vi "Write numAverages.vi"(8 "error in (no error)":errorcluster, 10 "numAverages":u16, 11 "CaptureSpectImage in":refnum<class "captureSpectImage.lvclass">) -> (0 "error out":errorcluster, 3 "CaptureSpectImage out":refnum<class "captureSpectImage.lvclass">)   [LabVIEW 2016, in "Commands.lvlib" / "captureSpectImage.lvclass"]
uses:
  captureSpectImage.lvclass
  captureSpectImage.lvclass/captureSpectImage.ctl
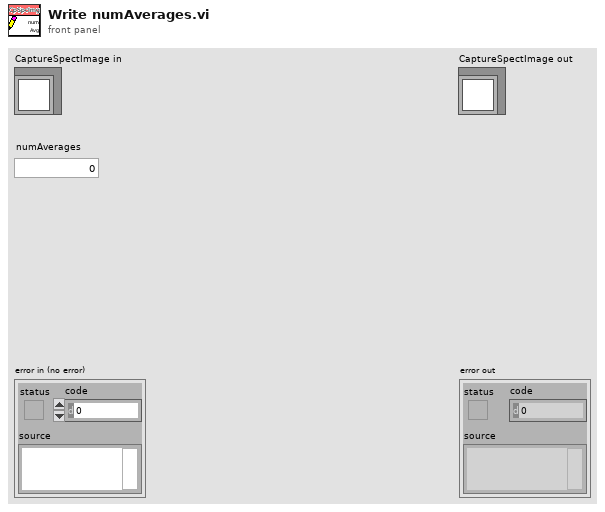
[diagram p1: front panel]
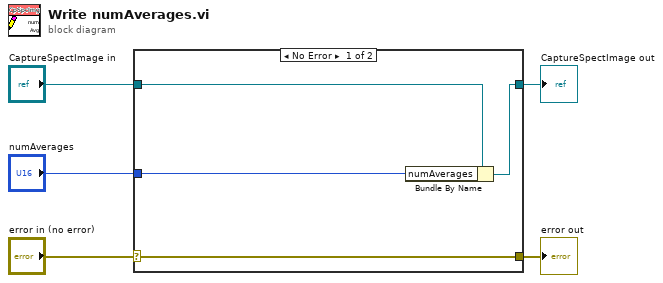
[diagram p0: block diagram]
diagram:
  n1 = case shown="No Error" "error in (no error)" {
    selector: "error in (no error)" -> [w9 w10]
    tunnel: [w9 w10] -> w4
    tunnel: [w7 w11] -> w2
    tunnel: "CaptureSpectImage in" -> [w8 w11]
    tunnel: "numAverages" -> [w6 _]
    frame No Error {
      n2 = Bundle By Name(cluster=w8, "numAverages"=w6) -> (w7:refnum<class "captureSpectImage.lvclass">)
    }
    frame Error {
    }
  }
  "error out" <- w4
  "CaptureSpectImage out" <- w2
